vi "Set Engine Base Pointer.vi"(10 "Engine Base Pointer":refnum<class "Pointer.lvclass">, 11 "Framework in":refnum<class "Framework.lvclass">) -> (3 "Framework out":refnum<class "Framework.lvclass">)   [LabVIEW 2017, in "DSF Core.lvlib" / "Framework.lvclass"]
uses:
  Framework.lvclass
  <vilib>/NI/Memory Manager/Classes/Pointer/Pointer.lvclass
  Framework.lvclass/Framework.ctl
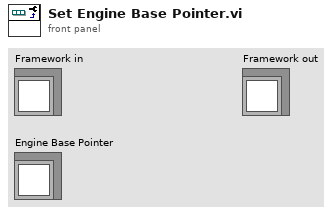
[diagram p1: front panel]
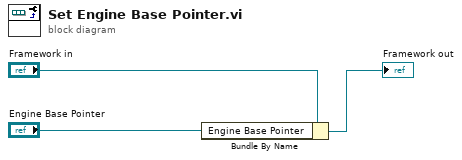
[diagram p0: block diagram]
diagram:
  n1 = Bundle By Name(cluster="Framework in", "Engine Base Pointer"="Engine Base Pointer") -> (→"Framework out":refnum<class "Framework.lvclass">)
